vi "SerialPort.Function_Write Data.vi"(5 "Timeout(ms)":i32=1000, 7 "Module Name":string="Serial Port", 8 "error in":errorcluster, 10 "Cmd":string, 11 "Q In":refnum<queue>) -> (0 "error out":errorcluster, 3 "Q Out":refnum<queue>)   [LabVIEW 2018]
uses:
  <vilib>/KATE/Queues/Q.Element.ctl
  <vilib>/KATE/Queues/Queue Utils.lvlib
panel:
  # "Serial Port Query"
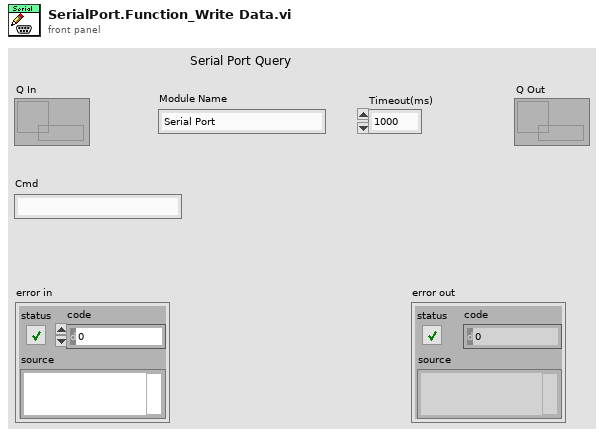
[diagram p1: front panel]
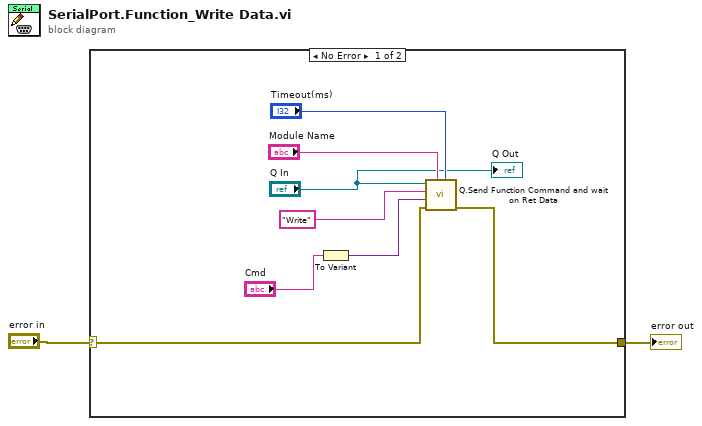
[diagram p0: block diagram]
diagram:
  n1 = case shown="No Error" "error in" {
    selector: "error in" -> [w7 w11]
    tunnel: [w6 w11] -> w1
    frame No Error {
      n2 = To Variant(anything="Cmd") -> (Variant=w5:variant)
      n3 = call <vilib>:"Q.Send Function Command and wait on Ret Data.vi"("Timeout(ms)"="Timeout(ms)", "Q Name"="Module Name", "error in"=w7, "Data1"=w5, "Cmd"="Write", "Q In"="Q In") -> ("error out"=w6:errorcluster)  [unwired: 4 in, 1 out]
      "Q Out" <- "Q In"
    }
    frame Error {
    }
  }
  "error out" <- w1
